vi "Start.vi"(9 "Team In":refnum<class "Team.lvclass">, 11 "MySquare in":refnum<class "MySquare.lvclass">) -> (1 "Team":refnum<class "Team.lvclass">, 3 "MySquare out":refnum<class "MySquare.lvclass">)   [LabVIEW 2020, in "DNattTeam.lvlib" / "MySquare.lvclass"]
uses:
  MySquare.lvclass
  SquareBattle/Team/Team.lvclass
  MyTeam/MyTeam.lvclass
  C:/dev/sol-squarebattle/SquareBattle/Team/Team.lvclass
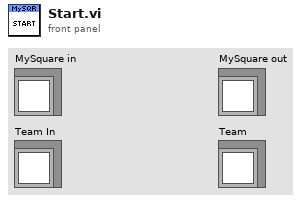
[diagram p1: front panel]
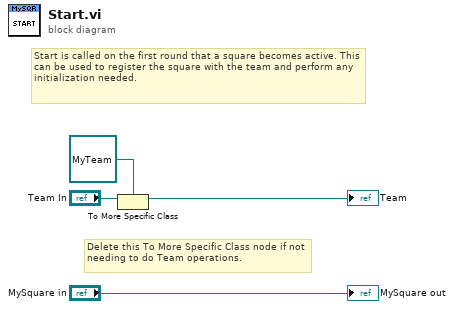
[diagram p0: block diagram]
diagram:
  # "Start is called on the first round that a square becomes active. This can be used to register the square with the team and perform any initialization needed."
  # "Delete this To More Specific Class node if not needing to do Team operations."
  n1 = To More Specific Class(target class=refnum<class "MyTeam.lvclass"> refnum ("SquareTeam.lvlib:MyTeam.lvclass"), reference="Team In") -> (specific class reference=→"Team":refnum<class "MyTeam.lvclass">)  [unwired: 1 in, 1 out]
  "MySquare out" <- "MySquare in"
